vi "Sort Ascending (multiple).vi"(8 "error in (no error)":errorcluster, 11 "Multiple XY-data in":cluster{"X-array":dbl[], "Y-array":dbl[]}[](array[cluster]) {"Y-array" format="%.2p"; "X-array" format="%.2p"}) -> (0 "error out":errorcluster, 3 "Multiple XY-data out":cluster{"X-array":dbl[], "Y-array":dbl[]}[](array[cluster]) {"Y-array" format="%.2p"; "X-array" format="%.2p"})   [LabVIEW 2016, in "xy_utilities.lvlib"]
uses:
  xy_utilities.lvlib
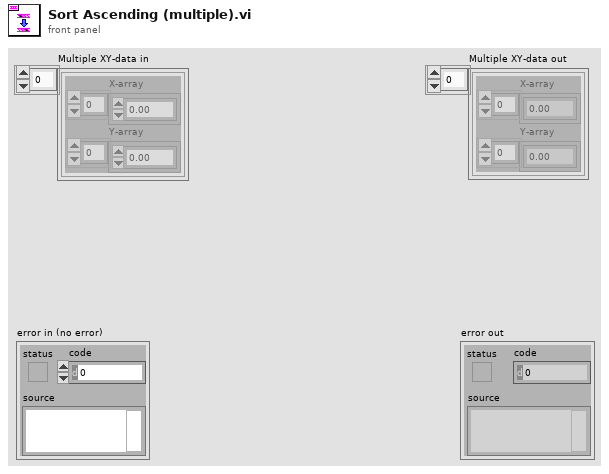
[diagram p1: front panel]
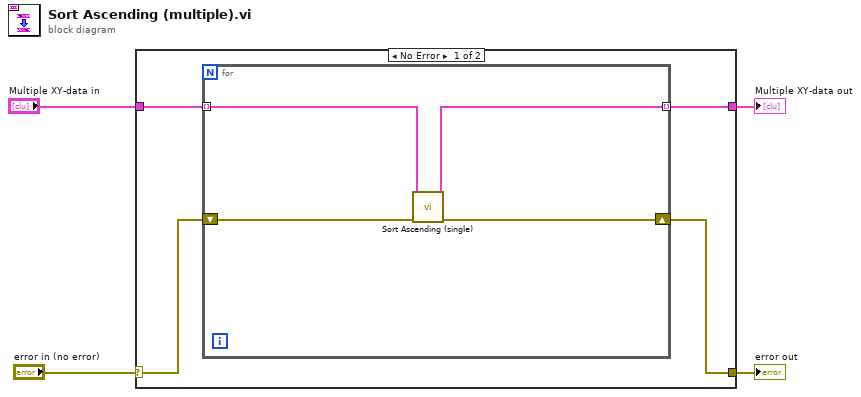
[diagram p0: block diagram]
diagram:
  n1 = case shown="No Error" "error in (no error)" {
    selector: "error in (no error)" -> [w5 w14]
    tunnel: [w6 w14] -> w3
    tunnel: "Multiple XY-data in" -> [w8 w13]
    tunnel: [w7 w13] -> w1
    frame No Error {
      n2 = for {
        tunnel: w8 -> [w12] mode=indexing
        tunnel: [w11] -> w7 mode=indexing
        shift-right: [w10] -> w6
        shift-left: w5 -> [w9]
        n3 = call "Sort Ascending (single).vi"("error in (no error)"=w9, "XY-data in"=w12) -> ("error out"=w10:errorcluster, "XY-data out"=w11:cluster{"X-array":dbl[], "Y-array":dbl[]})  [unwired: 8 in]
      }
    }
    frame Error {
    }
  }
  "error out" <- w3
  "Multiple XY-data out" <- w1
